vi "Draw_preview.vi"(7 "Draw_ops":T2, 8 "error in (no error)":errorcluster, 9 "Path":path, 11 "Picture ref":refnum<vi>) -> (0 "error out":errorcluster, 3 "Picture out":picture, 5 "Bus info":T1)   [LabVIEW 2010]
doc: "This orutine is used to draw a small scale preview of the system using the buscoords file provided.\n\nCreated by Davis Montenegro\n20-06-2016"
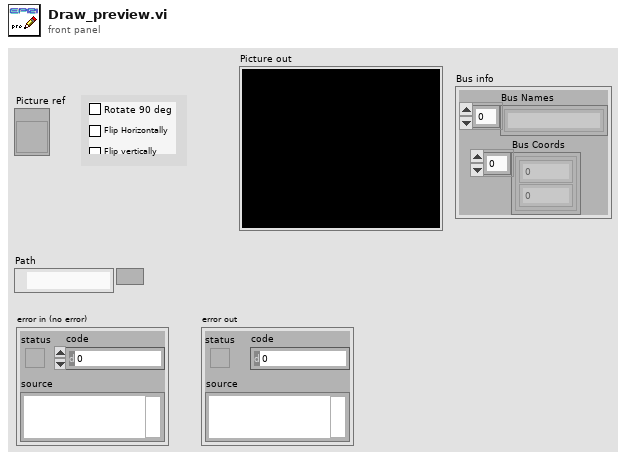
[diagram p1: front panel]
types:
  T1 = cluster{"Bus Names":string[], "Bus Coords":cluster{i32, i32}[]}
  T2 = cluster{"Rotate 90 deg":bool, "Flip Horizontally":bool, "Flip vertically":bool}
  T3 = typedef "LVBoundsTypeDef.ctl" = cluster{"Width":u32, "Height":u32}
  T4 = cluster{"Width":u16, "Style":enum32{"Solid", "Dash", "Dot", "DashDot", "DashDotDot"}}
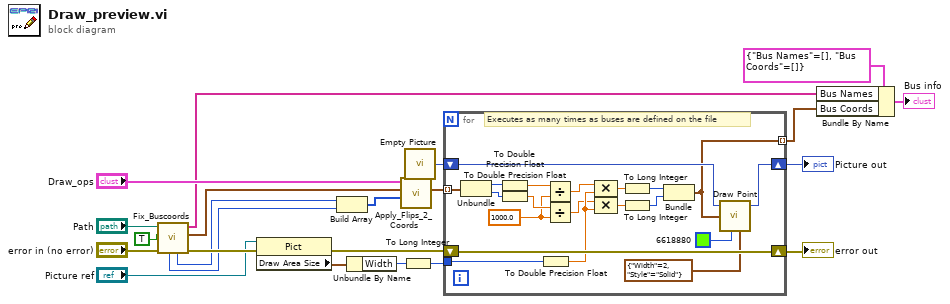
[diagram p0: block diagram]
diagram:
  n1 = call "Fix_Buscoords.vi"("error in (no error)"="error in (no error)", "Avoid screen ratio"=TRUE, "BusCoords Path"="Path") -> ("error out"=w19:errorcluster, "New positions"=w6:cluster{"X":i32, "Y":i32}[], "Bus_Name"=w3:string[], "Max X"=w11:i32, "Max Y"=w10:i32)  [unwired: 4 in]
  n2 = property on="Property Node" class="Pict"(reference="Picture ref", error in=w19) -> (error out=w16:errorcluster, "Draw Area Size"=w17:T3)  [unwired: 1 out]
  n3 = Build Array(w11, w10) -> (w7:i32[])
  n4 = Unbundle By Name(w17) -> ("Width"=w15:u32)
  n5 = call "Apply_Flips_2_Coords.vi"("Max Array"=w7, "Coords in"=w6, "Draw_ops"="Draw_ops") -> ("Coords out"=w8:cluster{"X":i32, "Y":i32}[])  [unwired: 8 in]
  n6 = To Long Integer(number=w15) -> (32bit integer=w9:i32)
  n7 = call "Empty Picture"() -> ("empty picture"=w14:picture)
  n8 = for {
    shift-right: [w42] -> w13
    shift-left: w16 -> [w42]
    tunnel: w9 -> [w37]
    shift-right: [w40] -> w12
    shift-left: w14 -> [w41]
    tunnel: w8 -> [w24] mode=indexing
    tunnel: [w23] -> w2 mode=indexing
    w30 = 1000.0 ("y")
    # "Executes as many times as buses are defined on the file"
    n9 = Unbundle(w24) -> ("X"=w28:i32, "Y"=w27:i32)
    n10 = To Double Precision Float(number=w28) -> (double precision float=w29:dbl)
    n11 = To Double Precision Float(number=w27) -> (double precision float=w35:dbl)
    n12 = To Double Precision Float(number=w37) -> (double precision float=w36:dbl)
    n13 = Divide(x=w29, y=w30) -> (x/y=w34:dbl)
    n14 = Divide(x=w35, y=w30) -> (x/y=w33:dbl)
    n15 = Compound Arithmetic op=MULTIPLY(w34, w36) -> (w32:dbl)
    n16 = Compound Arithmetic op=MULTIPLY(w33, w36) -> (w31:dbl)
    n17 = To Long Integer(number=w32) -> (32bit integer=w26:i32)
    n18 = To Long Integer(number=w31) -> (32bit integer=w25:i32)
    n19 = Bundle(w26, w25) -> (w23:cluster{i32, i32})  [unwired: 1 in]
    n20 = call <vilib>:"Draw Point.vi"("picture"=w41, "point(x,y)"=w23, "color(black)"=u32 6618880, "pen"=T4 {"Width"=2, "Style"=enum."Solid"}) -> ("new picture"=w40:picture)  [unwired: 5 in]
  }
  "error out" <- w13
  "Picture out" <- w12
  n21 = Bundle By Name(cluster=T1 {"Bus Names"=[], "Bus Coords"=[]}, "Bus Names"=w3, "Bus Coords"=w2) -> (→"Bus info":T1)
